vi "Set PlotImage Front.vi"(8 "error in":errorcluster, 10 "Plot Images:Front":picture, 11 "Base Graph in":refnum<class "Base Graph.lvclass">) -> (0 "error out":errorcluster, 3 "Base Graph out":refnum<class "Base Graph.lvclass">)   [LabVIEW 2025, in "Base Graph.lvclass"]
uses:
  Base Graph.lvclass
  Base Graph.lvclass/Base Graph.ctl
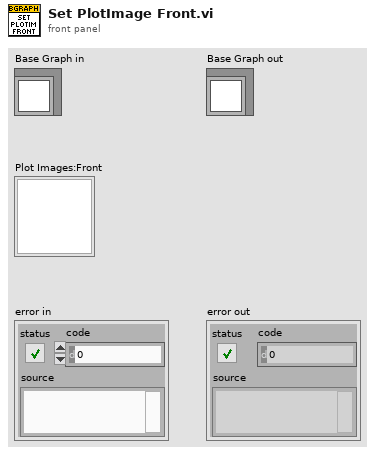
[diagram p1: front panel]
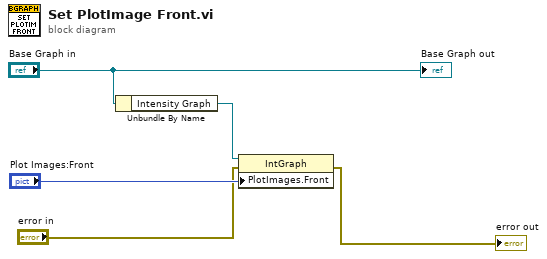
[diagram p0: block diagram]
diagram:
  n1 = Unbundle By Name("Base Graph in") -> ("Intensity Graph"=w3:refnum<vi>)
  n2 = property class="IntGraph"(reference=w3, error in="error in", "PlotImages.Front"="Plot Images:Front") -> (error out=→"error out":errorcluster)  [unwired: 1 out]
  "Base Graph out" <- "Base Graph in"
